vi "Close References.vi"(8 "error in (no error)":errorcluster, 11 "ZenGage v3.0 UI in":T1) -> (0 "error out":errorcluster)   [LabVIEW 2019, in "ZenGage v3.0 UI.lvclass"]
uses:
  ZenGage v3.0 UI.lvclass
  Type Definitions/Controls and Indicators/Select a part (combobox).ctl
  Type Definitions/Controls and Indicators/EDL control references.ctl
  Type Definitions/Controls and Indicators/Diagnostics control referencs.ctl
  Type Definitions/Controls and Indicators/Inspection control references.ctl
  Type Definitions/Controls and Indicators/General_Control references.ctl
  Type Definitions/Controls and Indicators/Controls and Indicators Cluster.ctl
  Type Definitions/General/Master sample references.ctl
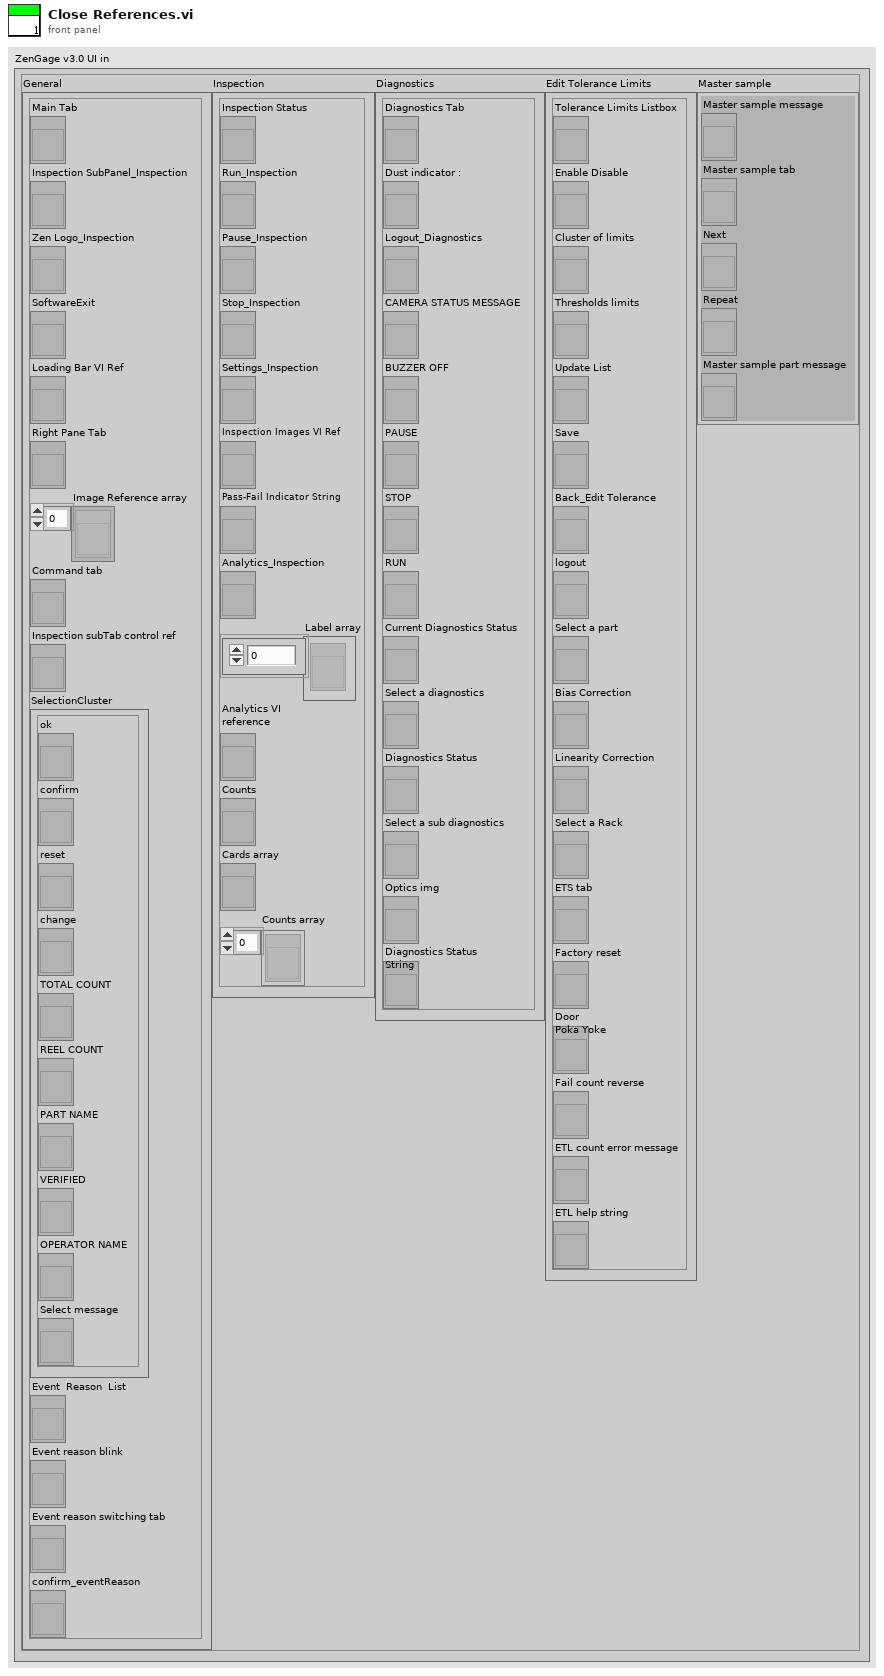
[diagram p1: front panel]
types:
  T1 = typedef "ZenGage v3.0 UI.lvclass/Controls and Indicators Cluster.ctl" = cluster{"General":T2, "Inspection":T3, "Diagnostics":T4, "Edit Tolerance Limits":T5, "Master sample":T6}
  T2 = typedef "ZenGage v3.0 UI.lvclass/General_Control references.ctl" = cluster{"Main Tab":refnum<vi>, "Inspection SubPanel_Inspection":refnum<vi>, "Zen Logo_Inspection":refnum<vi>, "SoftwareExit":refnum<vi>, "Loading Bar VI Ref":refnum<vi>, "Right Pane Tab":refnum<vi>, "Image Reference array":refnum<vi>[], "Command tab":refnum<vi>, "Inspection subTab control ref":refnum<vi>, "SelectionCluster":cluster{"ok":refnum<vi>, "confirm":refnum<vi>, "reset":refnum<vi>, "change":refnum<vi>, "TOTAL COUNT":refnum<vi>, "REEL COUNT":refnum<vi>, "PART NAME":refnum<vi>, "VERIFIED":refnum<vi>, "OPERATOR NAME":refnum<vi>, "Select message":refnum<vi>}, "Event  Reason  List":refnum<vi>, "Event reason blink":refnum<vi>, "Event reason switching tab":refnum<vi>, "confirm_eventReason":refnum<vi>}
  T3 = typedef "ZenGage v3.0 UI.lvclass/Inspection control references.ctl" = cluster{"Inspection Status":refnum<vi>, "Run_Inspection":refnum<vi>, "Pause_Inspection":refnum<vi>, "Stop_Inspection":refnum<vi>, "Settings_Inspection":refnum<vi>, "Inspection Images VI Ref":refnum<vi>, "Pass-Fail Indicator String":refnum<vi>, "Analytics_Inspection":refnum<vi>, "Label array":refnum<vi>[], "Analytics VI\nreference":refnum<vi>, "Counts":refnum<vi>, "Cards array":refnum<vi>, "Counts array":refnum<vi>[]}
  T4 = typedef "ZenGage v3.0 UI.lvclass/Diagnostics control referencs.ctl" = cluster{"Diagnostics Tab":refnum<vi>, "Dust indicator :":refnum<vi>, "Logout_Diagnostics":refnum<vi>, "CAMERA STATUS MESSAGE":refnum<vi>, "BUZZER OFF":refnum<vi>, "PAUSE":refnum<vi>, "STOP":refnum<vi>, "RUN":refnum<vi>, "Current Diagnostics Status":refnum<vi>, "Select a diagnostics":refnum<vi>, "Diagnostics Status":refnum<vi>, "Select a sub diagnostics":refnum<vi>, "Optics img":refnum<vi>, "Diagnostics Status\nString":refnum<vi>}
  T5 = typedef "ZenGage v3.0 UI.lvclass/EDL control references.ctl" = cluster{"Tolerance Limits Listbox":refnum<vi>, "Enable Disable":refnum<vi>, "Cluster of limits":refnum<vi>, "Thresholds limits":refnum<vi>, "Update List":refnum<vi>, "Save":refnum<vi>, "Back_Edit Tolerance":refnum<vi>, "logout":refnum<vi>, "Select a part":refnum<vi>, "Bias Correction":refnum<vi>, "Linearity Correction":refnum<vi>, "Select a Rack":refnum<vi>, "ETS tab":refnum<vi>, "Factory reset":refnum<vi>, "Door\nPoka Yoke":refnum<vi>, "Fail count reverse":refnum<vi>, "ETL count error message":refnum<vi>, "ETL help string":refnum<vi>}
  T6 = typedef "Master sample references.ctl" = cluster{"Master sample message":refnum<vi>, "Master sample tab":refnum<vi>, "Next":refnum<vi>, "Repeat":refnum<vi>, "Master sample part message":refnum<vi>}
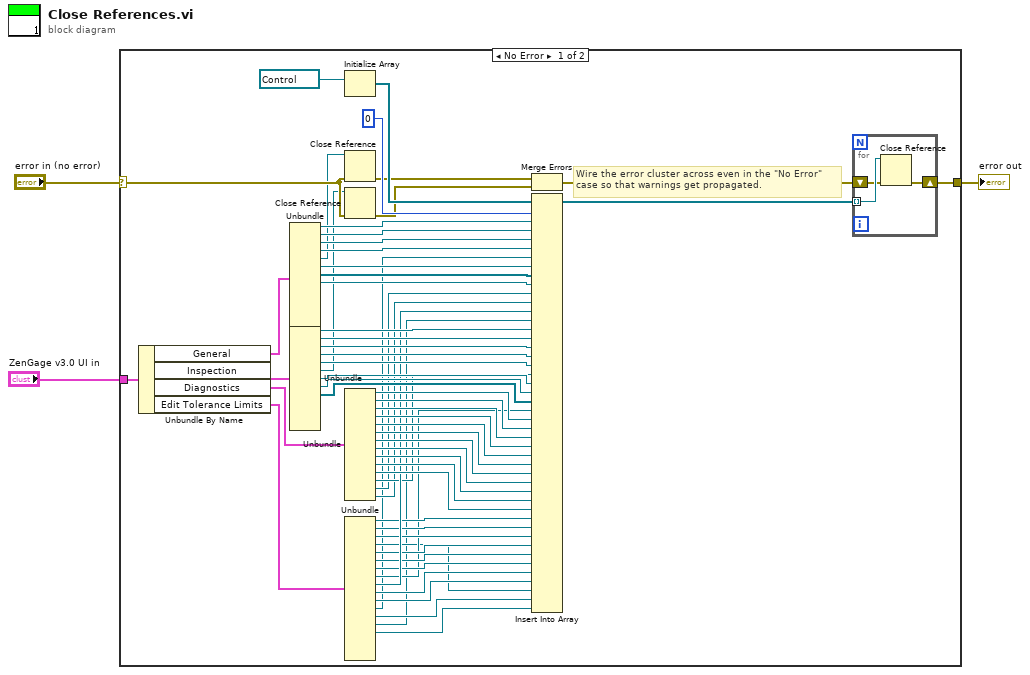
[diagram p0: block diagram]
diagram:
  n1 = case shown="No Error" "error in (no error)" {
    selector: "error in (no error)" -> [w26 w67]
    tunnel: [w14 w67] -> w2
    tunnel: "ZenGage v3.0 UI in" -> [w63 _]
    frame No Error {
      # "Wire the error cluster across even in the \"No Error\"\ncase so that warnings get propagated."
      n2 = Unbundle By Name(w63) -> ("General"=w62:T2, "Inspection"=w61:T3, "Diagnostics"=w60:T4, "Edit Tolerance Limits"=w25:T5)
      n3 = Unbundle(w62) -> ("Main Tab"=w56:refnum<vi>, "Inspection SubPanel_Inspection"=w55:refnum<vi>, "Zen Logo_Inspection"=w54:refnum<vi>, "SoftwareExit"=w53:refnum<vi>, "Loading Bar VI Ref"=w12:refnum<vi>, "Right Pane Tab"=w52:refnum<vi>, "Image Reference array"=w51:refnum<vi>[], "Command tab"=w50:refnum<vi>)  [unwired: 6 out]
      n4 = Unbundle(w61) -> ("Inspection Status"=w49:refnum<vi>, "Run_Inspection"=w48:refnum<vi>, "Pause_Inspection"=w47:refnum<vi>, "Stop_Inspection"=w46:refnum<vi>, "Settings_Inspection"=w45:refnum<vi>, "Inspection Images VI Ref"=w11:refnum<vi>, "Pass-Fail Indicator String"=w44:refnum<vi>, "Analytics_Inspection"=w43:refnum<vi>, "Label array"=w42:refnum<vi>[])  [unwired: 4 out]
      n5 = Initialize Array(refnum<vi> refnum ("Ctl Refnum")) -> (w58:refnum<vi>[])  [unwired: 1 in]
      n6 = Close Reference(reference=w12, error in (no error)=w26) -> (error out=w29:errorcluster)
      n7 = Close Reference(reference=w11, error in (no error)=w26) -> (error out=w28:errorcluster)
      n8 = Unbundle(w60) -> ("Diagnostics Tab"=w41:refnum<vi>, "Dust indicator :"=w40:refnum<vi>, "Logout_Diagnostics"=w39:refnum<vi>, "CAMERA STATUS MESSAGE"=w38:refnum<vi>, "BUZZER OFF"=w37:refnum<vi>, "PAUSE"=w36:refnum<vi>, "STOP"=w35:refnum<vi>, "RUN"=w34:refnum<vi>, "Current Diagnostics Status"=w33:refnum<vi>, "Select a diagnostics"=w32:refnum<vi>, "Diagnostics Status"=w31:refnum<vi>, "Select a sub diagnostics"=w10:refnum<vi>, "Optics img"=w9:refnum<vi>, "Diagnostics Status\nString"=w8:refnum<vi>)
      n9 = Unbundle(w25) -> ("Tolerance Limits Listbox"=w23:refnum<vi>, "Enable Disable"=w22:refnum<vi>, "Cluster of limits"=w21:refnum<vi>, "Thresholds limits"=w13:refnum<vi>, "Update List"=w20:refnum<vi>, "Save"=w19:refnum<vi>, "Back_Edit Tolerance"=w18:refnum<vi>, "logout"=w17:refnum<vi>, "Select a part"=w24:refnum<vi>, "Bias Correction"=w16:refnum<vi>, "Linearity Correction"=w15:refnum<vi>, "Select a Rack"=w7:refnum<vi>, "ETS tab"=w6:refnum<vi>, "Factory reset"=w5:refnum<vi>, "Door\nPoka Yoke"=w4:refnum<vi>)  [unwired: 3 out]
      n10 = Merge Errors(w29, w28) -> (w27:errorcluster)
      n11 = Insert Into Array(array=w58, index=0, new element #1=w56, new element #2=w55, new element #3=w54, new element #4=w53, new element #5=w7, new element #6=w52, new element #7=w51, new element #8=w50, new element #9=w9, new element #10=w8, new element #11=w24, new element #12=w5, new element #13=w49, new element #14=w48, new element #15=w47, new element #16=w46, new element #17=w45, new element #18=w10, new element #19=w44, new element #20=w43, new element #21=w42, new element #22=w17, new element #23=w41, new element #24=w40, new element #25=w39, new element #26=w38, new element #27=w37, new element #28=w36, new element #29=w35, new element #30=w34, new element #31=w33, new element #32=w32, new element #33=w31, new element #34=w23, new element #35=w22, new element #36=w21, new element #37=w20, new element #38=w19, new element #39=w18, new element #40=w16, new element #41=w15, new element #42=w13, new element #43=w6, new element #44=w4) -> (w30:refnum<vi>[])
      n12 = for {
        tunnel: w30 -> [w66] mode=indexing
        shift-right: [w64] -> w14
        shift-left: w27 -> [w65]
        n13 = Close Reference(reference=w66, error in (no error)=w65) -> (error out=w64:errorcluster)
      }
    }
    frame Error {
    }
  }
  "error out" <- w2
